vi "Get Event Log Count.vi"(8 "error in (no error)":errorcluster, 10 "Event Type":u16(ring) items=["All", "Error", "Warning", "Informational"], 11 "VISA resource name":refnum<visa-resource-name>) -> (0 "error out":errorcluster, 2 "Count":i32, 3 "VISA resource name out":refnum<visa-resource-name>)   [LabVIEW 2009, in "Keithley DMM7510.lvlib"]
doc: "This VI returns the number of events in the event log."
uses:
  Keithley DMM7510.lvlib
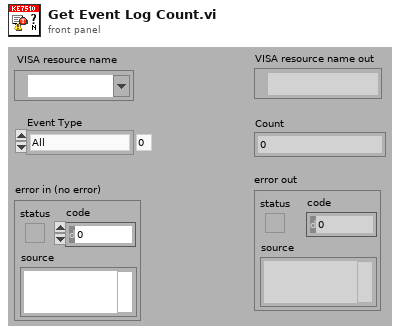
[diagram p1: front panel]
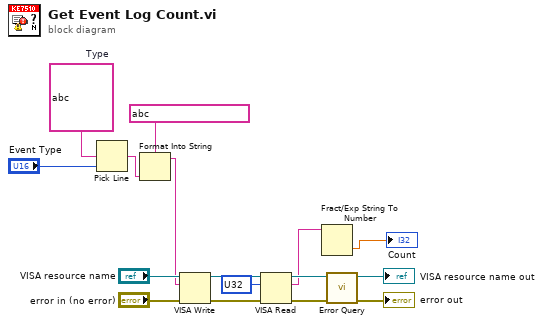
[diagram p0: block diagram]
diagram:
  w2 = string ?  # Type
  n1 = Pick Line(multi-line string=w2, line index="Event Type") -> (output string=w1:string)  [unwired: 1 in]
  n2 = Format Into String(format string=string ?, w1) -> (resulting string=w4:string)  [unwired: 2 in, 1 out]
  n3 = VISA Write(VISA resource name="VISA resource name", write buffer=w4, error in (no error)="error in (no error)") -> (VISA resource name out=w15:refnum<visa-resource-name>, error out=w16:errorcluster)  [unwired: 1 out]
  n4 = VISA Read(VISA resource name=w15, byte count=u32 ?, error in (no error)=w16) -> (VISA resource name out=w9:refnum<visa-resource-name>, read buffer=w7:string, error out=w8:errorcluster)  [unwired: 1 out]
  n5 = Fract/Exp String To Number(string=w7) -> (number=→"Count":dbl)  [unwired: 3 in, 1 out]
  n6 = call "Error Query.vi"("error in (no error)"=w8, "VISA resource name"=w9) -> ("error out"=→"error out":errorcluster, "VISA resource name out"=→"VISA resource name out":refnum<visa-resource-name>)  [unwired: 8 out]
